vi "tm_getarea.vi"(8 "error in (no error)":errorcluster, 11 "Handle in":u32) -> (0 "error out":errorcluster, 2 "Sub Region":T1, 3 "Handle out":u32)   [LabVIEW 2009]
uses:
  tmcamcon.dll
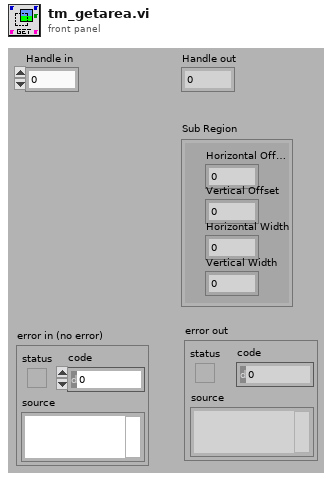
[diagram p1: front panel]
types:
  T1 = cluster{"Horizontal Offset":i32, "Vertical Offset":i32, "Horizontal Width":i32, "Vertical Width":i32}
  T2 = cluster{"sho":i32, "svo":i32, "shw":i32, "svw":i32}
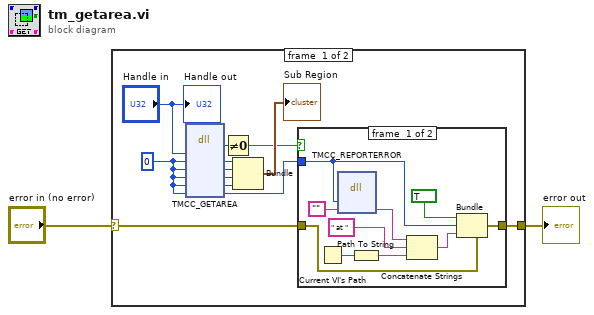
[diagram p0: block diagram]
diagram:
  n1 = case shown="No Error" "error in (no error)" {
    selector: "error in (no error)" -> [w4 w26]
    tunnel: [w3 w26] -> w1
    frame #0 {
      w13 = 0
      n2 = dll-call lib="tmcamcon.dll" fn="TMCC_GETAREA"("HDCAM"="Handle in", "sho"=w13, "svo"=w13, "shw"=w13, "svw"=w13, "Erval"=w13) -> (w14:u32, "sho"=w9:i32, "svo"=w10:i32, "shw"=w11:i32, "svw"=w8:i32, "Erval"=w5:i32)  [unwired: 4 in, 2 out]
      n3 = Not Equal To 0?(x=w14) -> (x != 0?=w6:bool)
      n4 = Bundle("sho"=w9, "svo"=w10, "shw"=w11, "svw"=w8) -> (→"Sub Region":T2)  [unwired: 1 in]
      n5 = case shown="False" w6 {
        tunnel: w4 -> [w24 w25]
        tunnel: [w23 w25] -> w3
        tunnel: w5 -> [w17 _]
        frame #0 {
          n6 = Current VI's Path() -> (path=w22:path)
          n7 = dll-call lib="tmcamcon.dll" fn="TMCC_REPORTERROR"("error"=w17, "buf"="") -> ("buf"=w16:string)  [unwired: 5 in, 2 out]
          n8 = Path To String(path=w22) -> (string=w18:string)
          n9 = Concatenate Strings(w16, " at ", w18) -> (w21:string)
          n10 = Bundle(cluster=w24, "status"=TRUE, "code"=w17, "source"=w21) -> (w23:errorcluster)
        }
        frame #1 {
        }
      }
      "Handle out" <- "Handle in"
    }
    frame #1 {
    }
  }
  "error out" <- w1
